vi "Periodic Tasks.vi"(8 "error in":errorcluster) -> ()   [LabVIEW 2015]
doc: "This VI runs in parallel to other tasks. It can contain as many user-defined periodic loops as you need. These can carry out PID or other sorts of timed response."
uses:
  Device Refnums.ctl
  Drive Base - Controlled Mode - TypeDef.ctl
  Drive Base Mode.ctl
  Shooter Control.ctl
  Arm Mode TypeDef.ctl
  <vilib>/Rock Robotics/WPI/Solenoid/WPI_SolenoidValue.ctl
  Projects/FRC Operator Interface Control Board/controlBoard_LabVIEW/LED_Output_TypeDef.ctl
  Projects/FRC Operator Interface Control Board/controlBoard_LabVIEW/PWM_Output_TypeDef.ctl
  <vilib>/Rock Robotics/WPI/CAN/TalonSRX/WPI_CANTalonSRX_APIControlMode.ctl
  <vilib>/Rock Robotics/WPI/Utilities/WPI_GetSetVariantRefNum.vi
  Global Variables.vi
  <vilib>/Rock Robotics/Network Tables/NT Write Number.vi
  <vilib>/Rock Robotics/Network Tables/NT Read Number.vi
  <vilib>/addons/control/pid/pid.llb/PID (DBL).vi
  <vilib>/Rock Robotics/Network Tables/NT Write Numeric Array.vi
  <vilib>/Rock Robotics/WPI/Solenoid/WPI_SolenoidSetEnum.vi
  <vilib>/Rock Robotics/Network Tables/NT Write String.vi
  <vilib>/Rock Robotics/Network Tables/NT Write Boolean.vi
  <vilib>/Rock Robotics/WPI/Ultrasonic/WPI_SonarMB1010DigitalRefNum Registry Get.vi
  <vilib>/Rock Robotics/WPI/Ultrasonic/WPI_SonarMB1010DigitalGetRange.vi
  ADIS16448-RoboRIO-Driver/trunk/LabVIEW/ADI MXP IMU/FRC ADI MXP IMU.lvlib
  <vilib>/addons/control/pid/NI_PID_pid.lvlib
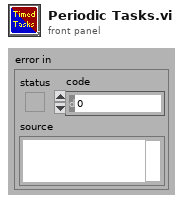
[diagram p1: front panel]
types:
  T1 = typedef "Device Refnums.ctl" = string
  T2 = typedef "Shooter Control.ctl" = cluster{"Fire":bool, "Open Claw":bool}
  T3 = typedef "Drive Base Mode.ctl" = enum16{"Disabled", "Controlled - Arcade", "Controlled - Tank", "Braked", "GRIP", "Encoder", "IMU", "Distance"}
  T4 = typedef "Drive Base - Controlled Mode - TypeDef.ctl" = cluster{"Drive Base Mode":T3, "Arcade":cluster{"y":dbl, "x":dbl}, "Tank":cluster{"Left":dbl, "Right":dbl}, "Target Encoder Value":cluster{"Left":dbl, "Right":dbl}, "Target IMU Angle":dbl, "Distance":dbl, "Target GRIP Area":dbl}
  T5 = typedef "WPI_EncoderDevRef.ctl" = cluster{"DevStatus":errorcluster, "EncoderIndex":T6, "CounterIndex":T7, "DistancePerCount":dbl, "Decoding Type":T8}
  T6 = typedef "FPGA_EncoderIdx.ctl" = enum8{"Enc 0", "Enc 1", "Enc 2", "Enc 3", "Enc 4", "Enc 5", "Enc 6", "Enc 7", "Invalid"}
  T7 = typedef "FPGA_CounterCtrSystemIndex.ctl" = enum8{"Ctr 0", "Ctr 1", "Ctr 2", "Ctr 3", "Ctr 4", "Ctr 5", "Ctr 6", "Ctr 7", "Invalid"}
  T8 = typedef "WPI_EncoderType.ctl" = enum16{"1x", "2x", "4x"}
  T9 = typedef "WPI_RobotDriveDevRef.ctl" = cluster{"DevStatus":errorcluster, "Motors[]":T10[], "Square Inputs":bool, "Max Output":dbl}
  T10 = typedef "WPI_MotorControlDeviceRef.ctl" = cluster{"DeviceStatus":errorcluster, "Type":T11, "PWM":cluster{"PWM Channel":T12, "DeadBand":T13}, "CAN":cluster{"Device Number":u8, "Control Mode":T14, "Semaphore":T15, "Max Vout":dbl, "TalonSRX Control Mode":T16}, "Invert":bool}
  T11 = typedef "WPI_MotorControlType.ctl" = enum16{"PWM", "CAN", "CANTalonSRX"}
  T12 = typedef "FPGA_DIOPWMChannel.ctl" = enum8{"PWM 0", "PWM 1", "PWM 2", "PWM 3", "PWM 4", "PWM 5", "PWM 6", "PWM 7", "PWM 8", "PWM 9", "PWM MXP 0", "PWM MXP 1", "PWM MXP 2", "PWM MXP 3", "PWM MXP 4", "PWM MXP 5", "PWM MXP 6", "PWM MXP 7", "PWM MXP 8", "PWM MXP 9", "Invalid"}
  T13 = typedef "WPI_PWMDeadband.ctl" = cluster{"Name":string, "maxPositivePwm":i32, "minPositivePwm":i32, "centerPwm":i32, "maxNegativePwm":i32, "minNegativePwm":i32, "angularRange":u16}
  T14 = typedef "WPI_CANJaguar_ControlMode.ctl" = enum8{"Percent VBus", "Current", "Speed", "Position", "Voltage"}
  T15 = typedef "Semaphore RefNum" = refnum<k1>
  T16 = typedef "WPI_CANTalonSRX_APIControlMode.ctl" = enum8{"Percent VBus", "Speed", "Position", "Slave", "Unchanged / Invalid", "Voltage Compensation", "Current", "Motion Profile"}
  T17 = typedef "WPI_SonarMB1010DigitalDeviceRef.ctl" = cluster{"CounterDevRef":T18, "Scaling factor (s/in)":dbl}
  T18 = typedef "WPI_CounterDevRef.ctl" = cluster{"DevStatus":errorcluster, "CntIndex":T7}
  T19 = typedef "FRC ADI MXP IMU.lvlib/WPI_AnalogDevicesIMUInterruptDevRef.ctl" = cluster{"SimpleGyroDevRef":T20, "InterruptRef":T22}
  T20 = typedef "FRC ADI MXP IMU.lvlib/WPI_AnalogDevicesIMUDevRef.ctl" = cluster{"DevStatus":errorcluster, "Handle":i32, "SPI Bus":T21, "Device Found":bool, "Sample Rate":dbl, "Device Ready":bool, "Yaw Axis":enum16{"X", "Y", "Z"}, "AHRS Algorithm":enum16{"Complementary", "Madgwick"}}
  T21 = typedef "spi_bus.ctl" = enum16{"SPI On-Board, CS0", "SPI On-Board, CS1", "SPI On-Board, CS2", "SPI On-Board, CS3", "SPI MXP", "Invalid"}
  T22 = typedef "WPI_InterruptRef.ctl" = cluster{"DevStatus":errorcluster, "InterruptIndex":T23}
  T23 = typedef "FPGA_InterruptIndex.ctl" = enum8{"0", "1", "2", "3", "4", "5", "6", "7", "Invalid"}
  T24 = typedef "WPI_AnalogChannelDevRef.ctl" = cluster{"DevStatus":errorcluster, "Analog Channel":T25}
  T25 = typedef "FPGA_AIChannel.ctl" = enum8{"AI 0", "AI 1", "AI 2", "AI 3", "AI MXP 0", "AI MXP 1", "AI MXP 2", "AI MXP 3", "Invalid"}
  T26 = typedef "Switch_Input_TypeDef.ctl" = cluster{"SW 0":bool, "SW 1":bool, "SW 2":bool, "SW 3":bool, "SW 4":bool, "SW 5":bool, "SW 6":bool, "SW 7":bool, "SW 8":bool, "SW 9":bool, "SW 10":bool, "SW 11":bool, "SW 12":bool, "SW 13":bool, "SW 14":bool, "SW 15":bool}
  T27 = typedef "GRIP Contours Report.ctl" = cluster{"area":dbl, "centerX":dbl, "centerY":dbl, "width":dbl, "height":dbl, "solidity":dbl}
  T28 = cluster{"proportional gain (Kc)":dbl, "integral time (Ti, min)":dbl, "derivative time (Td, min)":dbl}
  T29 = typedef "IMU AHRS TypeDef.ctl" = cluster{"Pitch":dbl, "Roll":dbl, "Yaw":dbl}
  T30 = typedef "WPI_SolenoidDevRef.ctl" = cluster{"DevStatus":errorcluster, "Pneumatics Control Module":u8, "Forward Solenoid Channel":T31, "Reverse Solenoid Channel":T31}
  T31 = typedef "WPI_SolenoidChannel.ctl" = enum8{"Solenoid 0", "Solenoid 1", "Solenoid 2", "Solenoid 3", "Solenoid 4", "Solenoid 5", "Solenoid 6", "Solenoid 7", "Invalid"}
  T32 = typedef "WPI_SolenoidValue.ctl" = enum16{"Off", "On", "Forward", "Reverse"}
  T33 = typedef "WPI_SwitchDevRef.ctl" = cluster{"DevStatus":errorcluster, "DIO Channel":T34, "CntIndex":T7, "Normally Closed":bool}
  T34 = typedef "FPGA_DIOChannel.ctl" = enum8{"DIO 0", "DIO 1", "DIO 2", "DIO 3", "DIO 4", "DIO 5", "DIO 6", "DIO 7", "DIO 8", "DIO 9", "DIO MXP 0", "DIO MXP 1", "DIO MXP 2", "DIO MXP 3", "DIO MXP 4", "DIO MXP 5", "DIO MXP 6", "DIO MXP 7", "DIO MXP 8", "DIO MXP 9", "DIO MXP 10", "DIO MXP 11", "DIO MXP 12", "DIO MXP 13", "DIO MXP 14", "DIO MXP 15", "Invalid"}
  T35 = typedef "Arm Mode TypeDef.ctl" = enum16{"Unknown", "Disabled", "Locked", "Shoot Batter", "Shoot Close", "Cross Defense", "Human Player Load", "Low Bar / Goal", "Manual"}
  T36 = typedef "Arm Notifier TypeDef.ctl" = cluster{"Arm Mode":T35, "Manual Arm Angle":dbl}
  T37 = typedef "PWM_Output_TypeDef.ctl" = cluster{"PWM 0":u8, "PWM 1":u8, "PWM 2":u8, "PWM 3":u8, "PWM 4":u8, "PWM 5":u8, "PWM 6":u8, "PWM 7":u8, "PWM 8":u8, "PWM 9":u8, "PWM 10":u8}
  T38 = typedef "LED_Output_TypeDef.ctl" = cluster{"LED 0":bool, "LED 1":bool, "LED 2":bool, "LED 3":bool, "LED 4":bool, "LED 5":bool, "LED 6":bool, "LED 7":bool, "LED 8":bool, "LED 9":bool, "LED 10":bool, "LED 11":bool, "LED 12":bool, "LED 13":bool, "LED 14":bool, "LED 15":bool}
  T39 = typedef "Arm Mode LEDs.ctl" = cluster{"Shoot Batter":bool, "Shoot Close":bool, "Shoot Far":bool, "Low Bar / Goal":bool, "Human Player Load":bool, "Manual":bool}
  T40 = typedef "Analog_Input_TypeDef.ctl" = cluster{"ANA 0":u8, "ANA 1":u8, "ANA 2":u8, "ANA 3":u8, "ANA 4":u8, "ANA 5":u8, "ANA 6":u8, "ANA 7":u8, "ANA 8":u8, "ANA 9":u8, "ANA 10":u8, "ANA 11":u8, "ANA 12":u8, "ANA 13":u8, "ANA 14":u8, "ANA 15":u8}
  T41 = typedef "Autonomous Mode.ctl" = enum16{"Off", "Cross Defense", "Shoot A/B", "Shoot C/D", "Shoot E"}
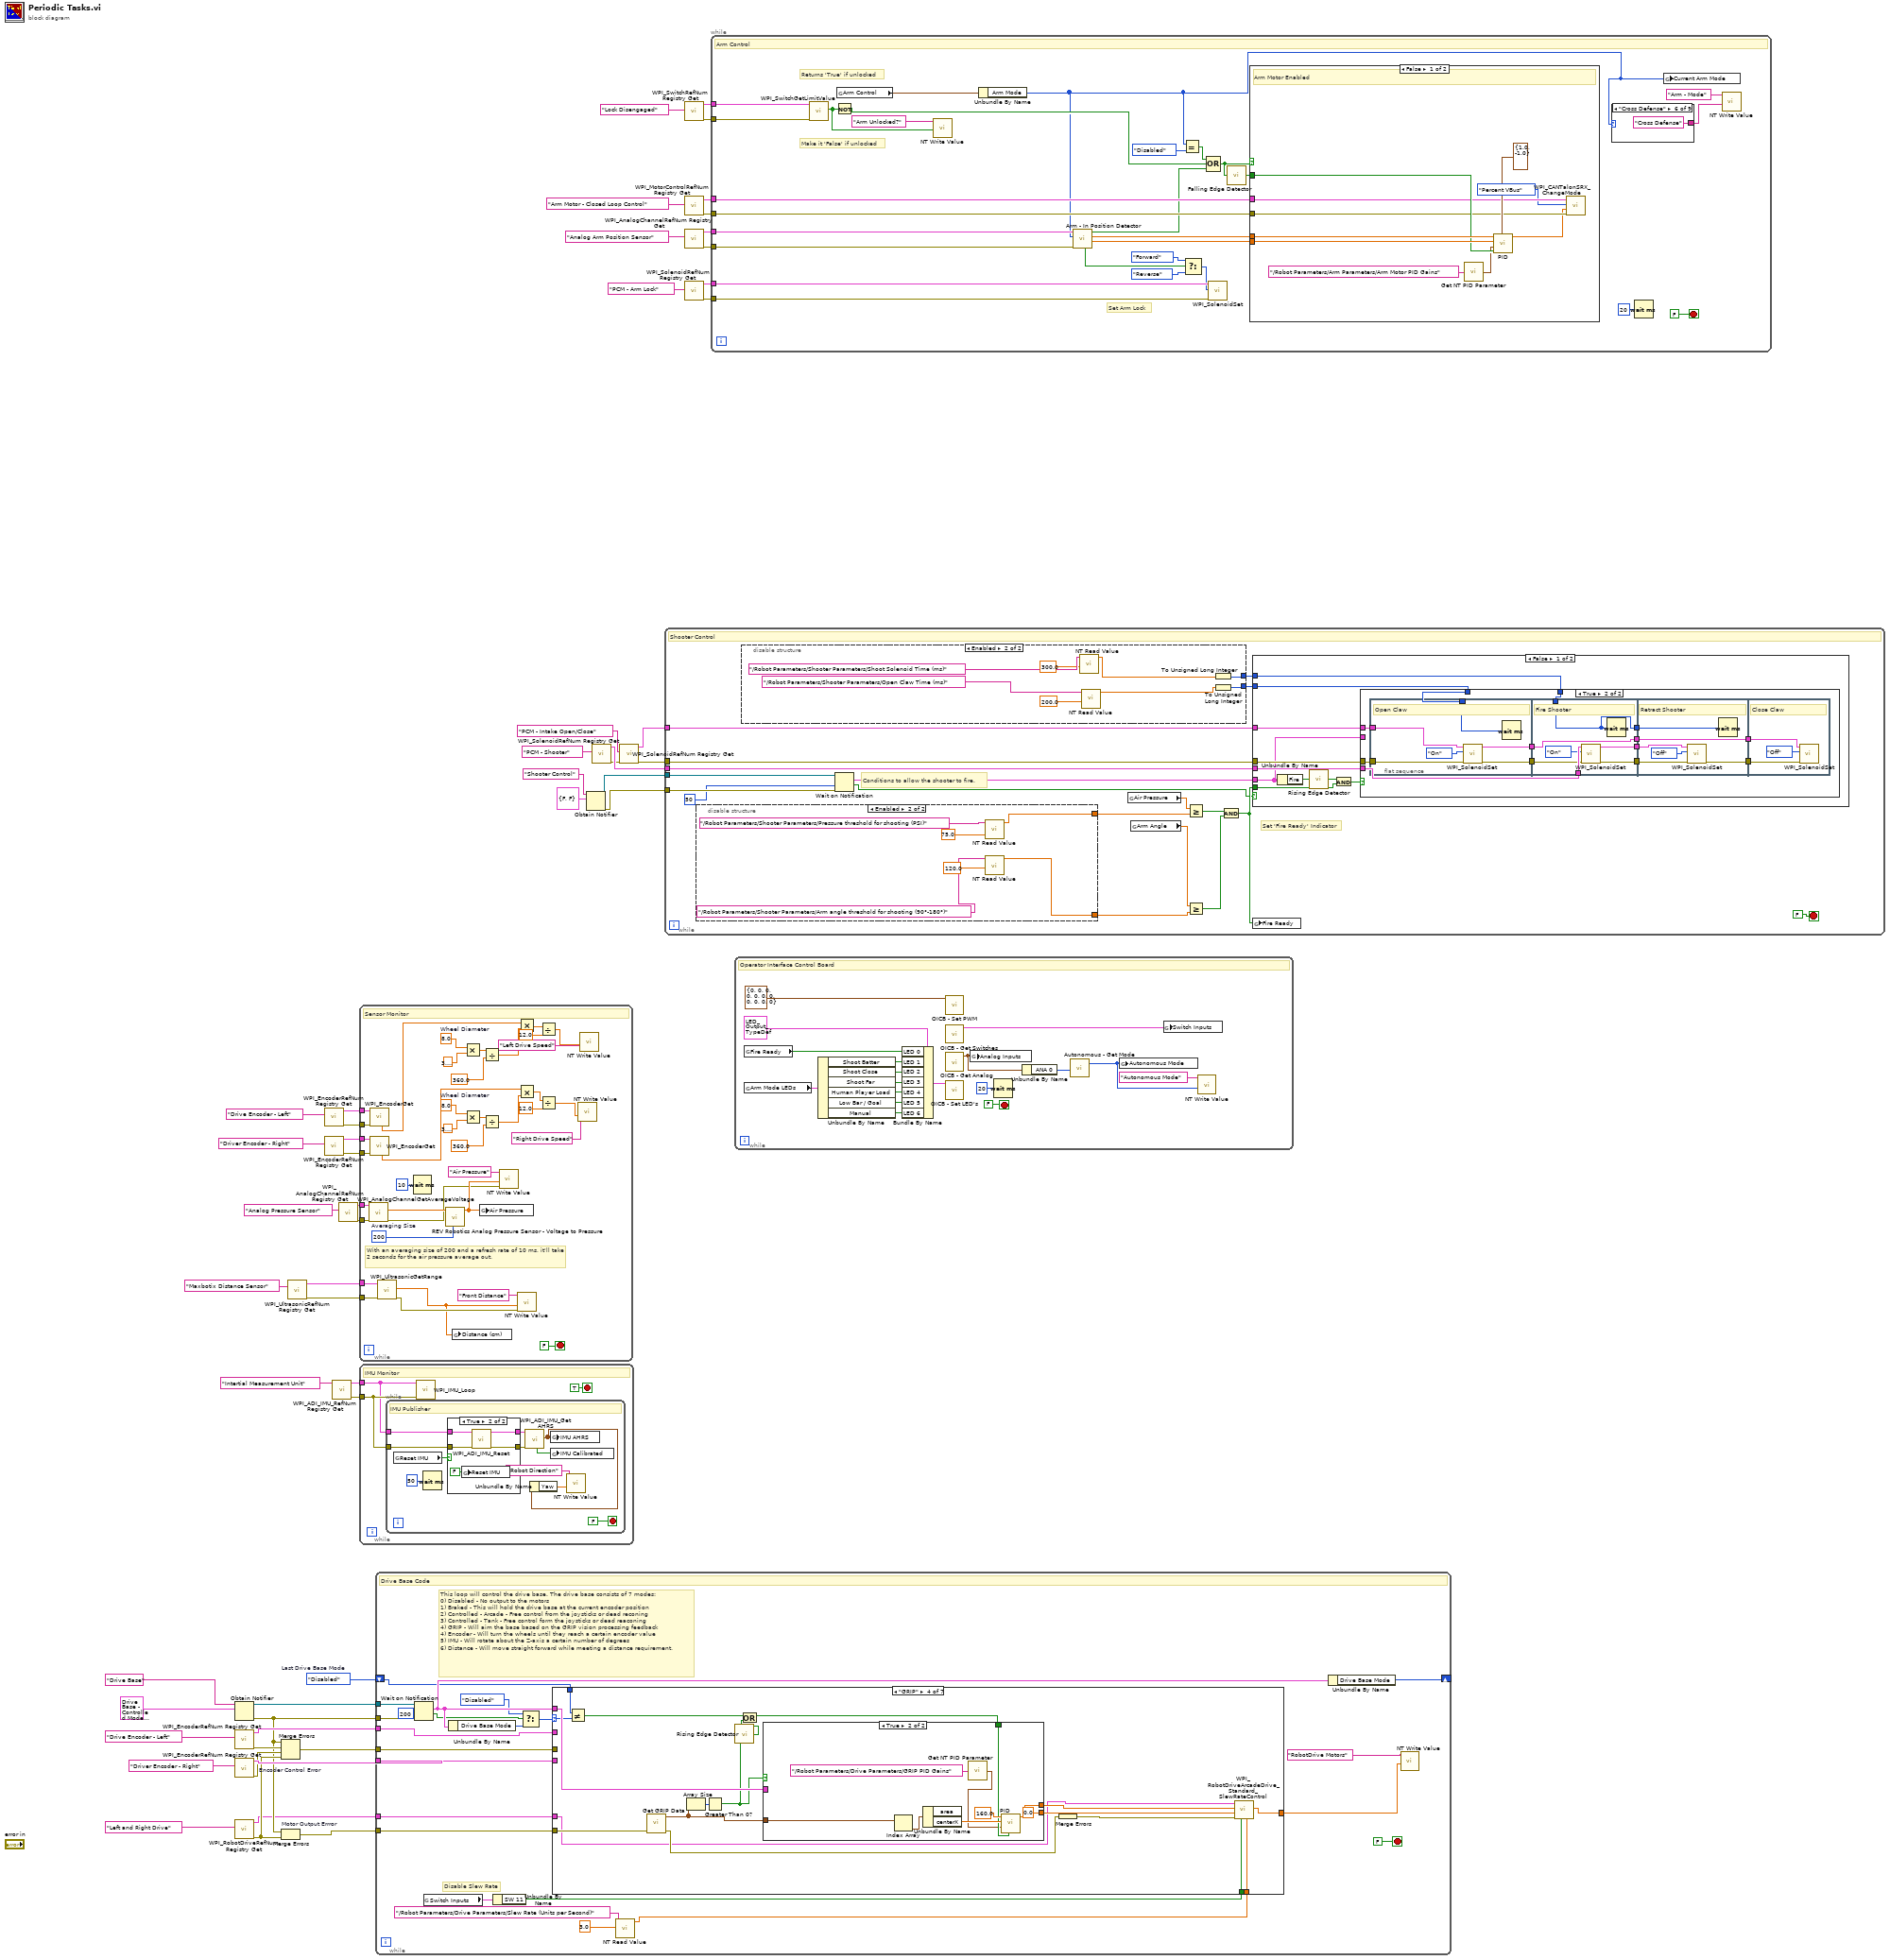
[diagram p0: block diagram]
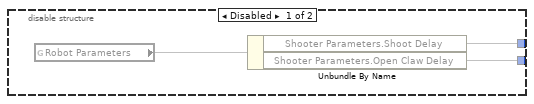
[diagram p3: hidden frame]
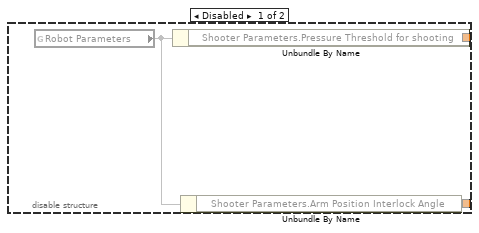
[diagram p4: hidden frame]
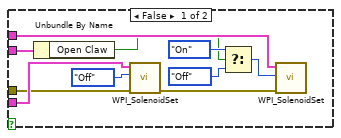
[diagram p5: hidden frame]
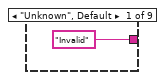
[diagram p7: hidden frame]
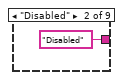
[diagram p8: hidden frame]
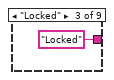
[diagram p9: hidden frame]
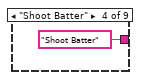
[diagram p10: hidden frame]
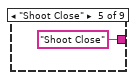
[diagram p11: hidden frame]
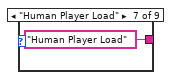
[diagram p12: hidden frame]
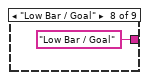
[diagram p13: hidden frame]
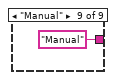
[diagram p14: hidden frame]
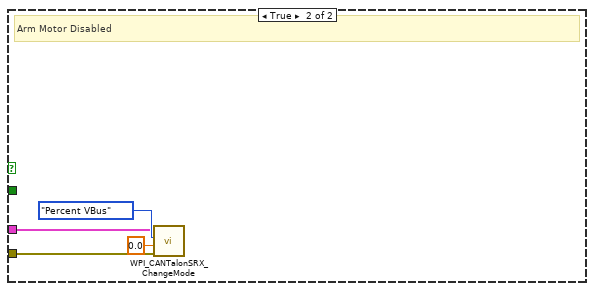
[diagram p15: hidden frame]
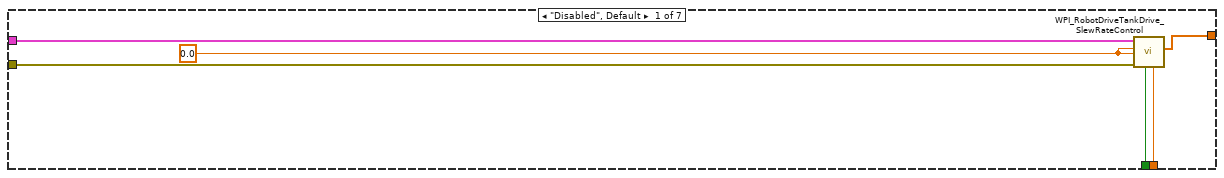
[diagram p16: hidden frame]
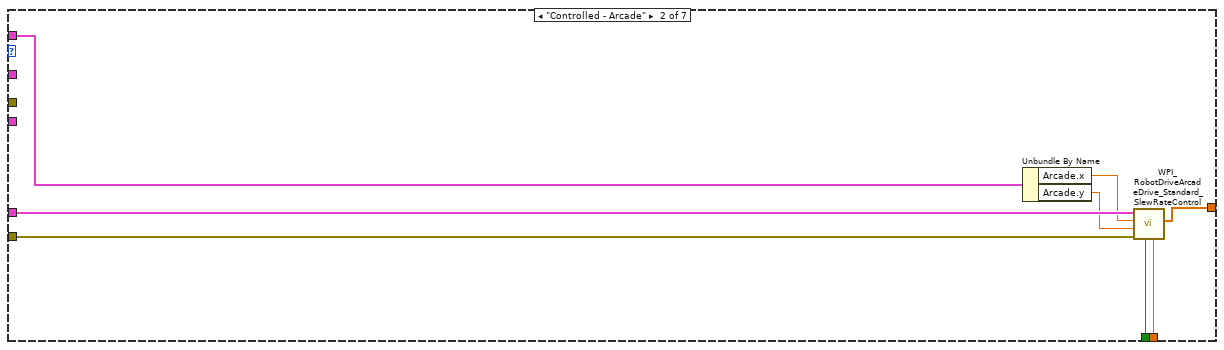
[diagram p17: hidden frame]
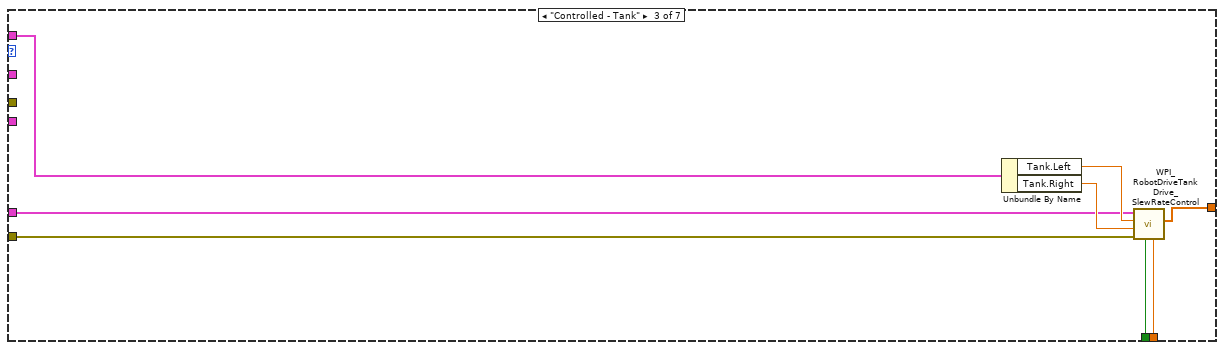
[diagram p18: hidden frame]
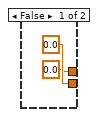
[diagram p19: hidden frame]
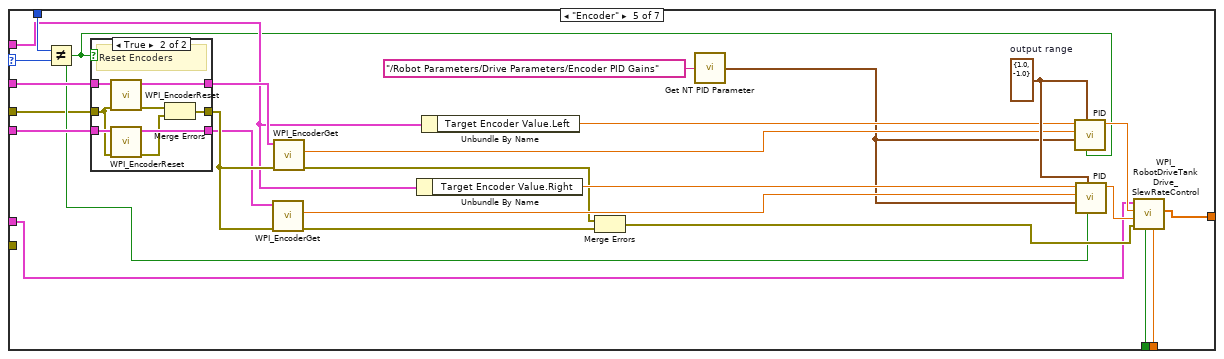
[diagram p20: hidden frame]
diagram:
  w37 = Drive_Base_Mode."Disabled"  # Last Drive Base Mode
  n1 = Obtain Notifier(name (unnamed)="Drive Base", notification data type=T4 {"Drive Base Mode"=enum."Disabled", "Arcade"={"y"=0.0, "x"=0.0}, "Tank"={"Left"=0.0, "Right"=0.0}, "Target Encoder Value"={"Left"=0.0, "Right"=0.0}, "Target IMU Angle"=0.0, "Distance"=0.0, "Target GRIP Area"=0.0}) -> (notifier out=w50:refnum<notifier>, error out=w40:errorcluster)  [unwired: 2 in, 1 out]
  n2 = call <vilib>:"WPI_EncoderRefNum Registry Get.vi"("refnum name"=T1 "Drive Encoder - Left" ("Device Name")) -> ("error out"=w44:errorcluster, "EncoderDevRef"=w47:T5)  [unwired: 9 in]
  n3 = call <vilib>:"WPI_EncoderRefNum Registry Get.vi"("refnum name"=T1 "Driver Encoder - Right" ("Device Name")) -> ("error out"=w43:errorcluster, "EncoderDevRef"=w46:T5)  [unwired: 9 in]
  n4 = call <vilib>:"WPI_RobotDriveRefNum Registry Get.vi"("refnum name"=T1 "Left and Right Drive" ("Device Name")) -> ("error out"=w41:errorcluster, "RobotDriveDevRef"=w39:T9)  [unwired: 1 in, 8 out]
  n5 = Merge Errors "Encoder Control Error"(w40, w44, w43, w41) -> (w42:errorcluster)
  n6 = Merge Errors "Motor Output Errror"(w40, w41) -> (w38:errorcluster)
  n7 = call-poly <vilib>:"WPI_UltrasonicRefNum Registry Get.vi"("refnum name"=T1 "Maxbotix Distance Sensor" ("Device Name")) -> ("error out"=w7:errorcluster, "SonarMB1010DigitalDevRef"=w8:T17)  [unwired: 9 in]
  n8 = call <vilib>:"WPI_EncoderRefNum Registry Get.vi"("refnum name"=T1 "Drive Encoder - Left" ("Device Name")) -> ("error out"=w3:errorcluster, "EncoderDevRef"=w4:T5)  [unwired: 9 in]
  n9 = call <vilib>:"WPI_EncoderRefNum Registry Get.vi"("refnum name"=T1 "Driver Encoder - Right" ("Device Name")) -> ("error out"=w1:errorcluster, "EncoderDevRef"=w2:T5)  [unwired: 9 in]
  n10 = call "WPI_ADI_IMU_RefNum Registry Get.vi"("refnum name"=T1 "Intertial Measurement Unit" ("Device Name")) -> ("error out"=w13:errorcluster, "ADI IMU Interrupt DevRef"=w12:T19)  [unwired: 9 in]
  n11 = call <vilib>:"WPI_AnalogChannelRefNum Registry Get.vi"("refnum name"=T1 "Analog Pressure Sensor" ("Device Name")) -> ("error out"=w18:errorcluster, "AIDeviceRef"=w19:T24)  [unwired: 9 in]
  n12 = while {
    tunnel: w19 -> [w87]
    tunnel: w18 -> [w86]
    tunnel: w8 -> [w82]
    tunnel: w7 -> [w83]
    tunnel: w4 -> [w77]
    tunnel: w3 -> [w76]
    tunnel: w2 -> [w75]
    tunnel: w1 -> [w74]
    stop <- FALSE stop-if-true
    w67 = 8.0  # Wheel Diameter
    w70 = 8.0  # Wheel Diameter
    w85 = 200  # Averaging Size
    # "With an averaging size of 200 and a refresh rate of 10 ms, it'll take 2 seconds for the air pressure average out."
    # "Sensor Monitor"
    n13 = call <vilib>:"WPI_AnalogChannelGetAverageVoltage.vi"("error in (no error)"=w86, "AIDeviceRef"=w87) -> ("error out"=w79:errorcluster, "Voltage"=w89:dbl)  [unwired: 7 in, 1 out]
    n14 = call <vilib>:"WPI_EncoderGet.vi"("error in (no error)"=w76, "EncoderDevRef"=w77) -> ("Rate"=w63:dbl)  [unwired: 4 in, 5 out]
    n15 = call <vilib>:"WPI_EncoderGet.vi"("error in (no error)"=w74, "EncoderDevRef"=w75) -> ("Rate"=w62:dbl)  [unwired: 4 in, 5 out]
    n16 = call-poly <vilib>:"WPI_UltrasonicGetRange.vi"("error in"=w83, "SonarMB1010DigitalDevRef"=w82) -> ("error out"=w80:errorcluster, "Distance"=w78:dbl)  [unwired: 7 in, 1 out]
    n17 = Wait (ms)(milliseconds to wait=u32 10) -> ()  [unwired: 1 out]
    n18 = call "REV Robotics Analog Pressure Sensor - Voltage to Pressure.vi"("Averaging Size"=w85, "Voltage (V)"=w89) -> ("Pressure (PSI)"=w84:dbl)  [unwired: 7 in]
    n19 = global write "Global Variables.vi" "Distance (cm)"(w78) -> ()
    n20 = Multiply(x=w67, y=3.141592653589793) -> (x*y=w66:dbl)
    n21 = Multiply(x=w70, y=3.141592653589793) -> (x*y=w71:dbl)
    n22 = global write "Global Variables.vi" "Air Pressure"(w84) -> ()
    n23 = Divide(x=w66, y=360.0) -> (x/y=w64:dbl)
    n24 = Divide(x=w71, y=360.0) -> (x/y=w73:dbl)
    n25 = call-poly <vilib>:"NT Write Value.vi"("error in"=w79, "Numeric"=w84, "Name"="Air Pressure") -> ()  [unwired: 8 in, 1 out]
    n26 = call-poly <vilib>:"NT Write Value.vi"("error in"=w80, "Numeric"=w78, "Name"="Front Distance") -> ()  [unwired: 8 in, 1 out]
    n27 = Multiply(x=w63, y=w64) -> (x*y=w61:dbl)
    n28 = Multiply(x=w62, y=w73) -> (x*y=w58:dbl)
    n29 = Divide(x=w61, y=12.0) -> (x/y=w54:dbl)
    n30 = Divide(x=w58, y=12.0) -> (x/y=w55:dbl)
    n31 = call-poly <vilib>:"NT Write Value.vi"("Numeric"=w55, "Name"="Right Drive Speed") -> ()  [unwired: 9 in, 1 out]
    n32 = call-poly <vilib>:"NT Write Value.vi"("Numeric"=w54, "Name"="Left Drive Speed") -> ()  [unwired: 9 in, 1 out]
  }
  n33 = while {
    tunnel: w13 -> [w94]
    tunnel: w12 -> [w93]
    stop <- TRUE stop-if-true
    # "IMU Monitor"
    n34 = while {
      tunnel: w94 -> [w101]
      tunnel: w93 -> [w102]
      stop <- FALSE stop-if-true
      # "IMU Publisher"
      n35 = global read "Global Variables.vi" "Reset IMU"() -> (w103:bool)
      n36 = Wait (ms)(milliseconds to wait=u32 50) -> ()  [unwired: 1 out]
      n37 = case shown="True" w103 {
        tunnel: w102 -> [w107 w111]
        tunnel: w101 -> [w106 w110]
        tunnel: [w107 w109] -> w99
        tunnel: [w106 w108] -> w98
        frame False {
        }
        frame True {
          n38 = global write "Global Variables.vi" "Reset IMU"(FALSE ("Reset IMU")) -> ()
          n39 = call "WPI_ADI_IMU_Reset.vi"("error in"=w110, "ADI IMU Interrupt DevRef"=w111) -> ("error out"=w108:errorcluster, "ADI IMU Interrupt DevRef Out"=w109:T19)  [unwired: 8 in]
        }
      }
      n40 = call "WPI_ADI_IMU_Get AHRS.vi"("error in"=w98, "ADI IMU Interrupt DevRef"=w99) -> ("IMU AHRS"=w96:cluster{"Pitch":dbl, "Roll":dbl, "Yaw":dbl}, "Sensor Ready Out"=w100:bool)  [unwired: 5 in, 3 out]
      n41 = Unbundle By Name(w96) -> ("Yaw"=w95:dbl)
      n42 = global write "Global Variables.vi" "IMU AHRS"(w96) -> ()
      n43 = global write "Global Variables.vi" "IMU Calibrated"(w100) -> ()
      n44 = call-poly <vilib>:"NT Write Value.vi"("Numeric"=w95, "Name"="Robot Direction") -> ()  [unwired: 9 in, 1 out]
    }
    n45 = call "WPI_IMU_Loop.vi"("error in"=w94, "ADI IMU Interrupt DevRef"=w93) -> ()  [unwired: 8 in, 2 out]
  }
  n46 = while {
    tunnel: w39 -> [w134]
    tunnel: w50 -> [w133]
    tunnel: w40 -> [w132]
    tunnel: w47 -> [w131]
    tunnel: w46 -> [w130]
    tunnel: w42 -> [w128]
    tunnel: w38 -> [w129]
    shift-right: [w127] -> _
    shift-left: w37 -> [w125]
    stop <- FALSE stop-if-true
    # "Disable Slew Rate"
    # "This loop will control the drive base. The drive base consists of 7 modes:\n0) Disabled - No output to the motors\n1) Braked - This will hold the drive base at the current encoder position\n2) Controlled - Arcade - Free control from the joysticks or dead reconing\n3) Controlled - Tank - Free control form the joysticks or dead reaconing\n4) GRIP - Will aim the base based on the GRIP vision processing feedback\n4) Encoder - Will turn the wheels until they reach a certain encoder value\n5) IMU - Will rotate about the Z-axis a certain number of degrees\n6) Distance - Will move straight forward while meeting a distance requirement."
    # "Drive Base Code"
    n47 = Wait on Notification(notifier=w133, timeout in ms (-1)=200, error in (no error)=w132) -> (notification=w126:T4, timed out?=w123:bool)  [unwired: 1 in, 2 out]
    n48 = global read "Global Variables.vi" "Switch Inputs"() -> (w117:T26)
    n49 = Unbundle By Name(w126) -> ("Drive Base Mode"=w122:T3)
    n50 = Unbundle By Name(w117) -> ("SW 11"=w116:bool)
    n51 = Select(t=Drive_Base_Mode."Disabled", s=w123, f=w122) -> (s? t:f=w120:T3)
    n52 = call-poly <vilib>:"NT Read Value.vi"("Default Value"=3.0, "Name"="/Robot Parameters/Drive Parameters/Slew Rate (Units per Second)") -> ("Numeric"=w115:dbl)  [unwired: 8 in, 1 out]
    n53 = case shown="\"GRIP\"" w120 {
      selector: w120 -> [_ _ _ w172 w211 w241 w260]
      tunnel: w134 -> [w141 w149 w154 w160 w194 w238 w259]
      tunnel: w126 -> [_ w147 w153 w175 w198 w237 _]
      tunnel: w131 -> [_ _ _ _ w210 _ w265]
      tunnel: w130 -> [_ _ _ _ w209 _ w264]
      tunnel: w129 -> [w139 w148 w155 w174 _ w236 _]
      tunnel: w128 -> [_ _ _ _ w191 _ w257]
      tunnel: w125 -> [_ _ _ w171 w212 w240 w261]
      tunnel: [w138 w144 w152 w164 w193 w231 w258] -> w118
      tunnel: w116 -> [w137 w143 w151 w159 w190 w227 w256]
      tunnel: w115 -> [w136 w142 w150 w158 w189 w226 w255]
      frame "Disabled", Default {
        w140 = 0.0
        n54 = call "WPI_RobotDriveTankDrive_SlewRateControl.vi"("Slew Rate (Unit/Sec)"=w136, "Disable Slew"=w137, "error in (no error)"=w139, "Right axis value"=w140, "Left axis value"=w140, "RobotDriveDevRef"=w141) -> ("Motor Values"=w138:dbl[])  [unwired: 3 in, 2 out]
      }
      frame "Controlled - Arcade" {
        n55 = Unbundle By Name(w147) -> ("Arcade.x"=w145:dbl, "Arcade.y"=w146:dbl)
        n56 = call "WPI_RobotDriveArcadeDrive_Standard_SlewRateControl.vi"("Slew Rate (Unit/Sec)"=w142, "Disable Slew"=w143, "error in (no error)"=w148, "Y axis value"=w146, "X axis value"=w145, "RobotDriveDevRef"=w149) -> ("Motor Values"=w144:dbl[])  [unwired: 3 in, 2 out]
      }
      frame "Controlled - Tank" {
        n57 = Unbundle By Name(w153) -> ("Tank.Left"=w157:dbl, "Tank.Right"=w156:dbl)
        n58 = call "WPI_RobotDriveTankDrive_SlewRateControl.vi"("Slew Rate (Unit/Sec)"=w150, "Disable Slew"=w151, "error in (no error)"=w155, "Right axis value"=w156, "Left axis value"=w157, "RobotDriveDevRef"=w154) -> ("Motor Values"=w152:dbl[])  [unwired: 3 in, 2 out]
      }
      frame "GRIP" {
        n59 = Not Equal?(x=w171, y=w172) -> (x != y?=w170:bool)
        n60 = call "Get GRIP Data.vi"("error in (no error)"=w174) -> ("error out"=w173:errorcluster, "ContoursReport"=w169:T27[])  [unwired: 8 in, 1 out]
        n61 = Array Size(array=w169) -> (size(s)=w168:i32)
        n62 = Greater Than 0?(x=w168) -> (x > 0?=w167:bool)
        n63 = call "Rising Edge Detector.vi"("Input"=w167) -> ("Rising Edge Detected"=w165:bool)
        n64 = Or(x=w170, y=w165) -> (x .or. y?=w166:bool)
        n65 = case shown="True" w167 {
          tunnel: w175 -> [_ _]
          tunnel: w166 -> [_ w183]
          tunnel: [0.0 ("output") 0.0 ("output")] -> w162
          tunnel: [0.0 ("output") w182] -> w163
          tunnel: w169 -> [_ w181]
          frame False {
          }
          frame True {
            n66 = Index Array(array=w181) -> (element=w186:T27)  [unwired: 1 in]
            n67 = Unbundle By Name(w186) -> ("centerX"=w185:dbl)  [unwired: 1 out]
            n68 = call "Get NT PID Parameter.vi"("NT Path"="/Robot Parameters/Drive Parameters/GRIP PID Gains") -> ("PID Gains"=w178:T28)
            n69 = call-poly <vilib>:"PID.vi"("reinitialize? (F)"=w183, "PID gains"=w178, "process variable"=w185, "setpoint"=160.0) -> ("output"=w182:dbl)  [unwired: 6 in, 1 out]
          }
        }
        n70 = Merge Errors(w173) -> (w161:errorcluster)
        n71 = call "WPI_RobotDriveArcadeDrive_Standard_SlewRateControl.vi"("Slew Rate (Unit/Sec)"=w158, "Disable Slew"=w159, "error in (no error)"=w161, "Y axis value"=w162, "X axis value"=w163, "RobotDriveDevRef"=w160) -> ("Motor Values"=w164:dbl[])  [unwired: 3 in, 2 out]
      }
      frame "Encoder" {
        w208 = cluster{"output high":dbl, "output low":dbl} {"output high"=1.0, "output low"=-1.0}  # output range
        n72 = Not Equal?(x=w212, y=w211) -> (x != y?=w192:bool)
        n73 = case shown="True" w192 {
          tunnel: w210 -> [w215 w223]
          tunnel: w209 -> [w214 w222]
          tunnel: [w215 w221] -> w206
          tunnel: [w214 w220] -> w205
          tunnel: [w213 w219] -> w207
          tunnel: w191 -> [w213 w216]
          frame False {
          }
          frame True {
            # "Reset Encoders"
            n74 = call <vilib>:"WPI_EncoderReset.vi"("error in (no error)"=w216, "EncoderDevRef"=w223) -> ("error out"=w218:errorcluster, "EncoderDevRef"=w221:T5)  [unwired: 8 in]
            n75 = call <vilib>:"WPI_EncoderReset.vi"("error in (no error)"=w216, "EncoderDevRef"=w222) -> ("error out"=w217:errorcluster, "EncoderDevRef"=w220:T5)  [unwired: 8 in]
            n76 = Merge Errors(w218, w217) -> (w219:errorcluster)
          }
        }
        n77 = call <vilib>:"WPI_EncoderGet.vi"("error in (no error)"=w207, "EncoderDevRef"=w205) -> ("error out"=w196:errorcluster, "Distance"=w203:dbl)  [unwired: 4 in, 4 out]
        n78 = call <vilib>:"WPI_EncoderGet.vi"("error in (no error)"=w207, "EncoderDevRef"=w206) -> ("error out"=w197:errorcluster, "Distance"=w204:dbl)  [unwired: 4 in, 4 out]
        n79 = Unbundle By Name(w198) -> ("Target Encoder Value.Right"=w199:dbl)
        n80 = Unbundle By Name(w198) -> ("Target Encoder Value.Left"=w200:dbl)
        n81 = Merge Errors(w197, w196) -> (w195:errorcluster)
        n82 = call "Get NT PID Parameter.vi"("NT Path"="/Robot Parameters/Drive Parameters/Encoder PID Gains") -> ("PID Gains"=w187:T28)
        n83 = call-poly <vilib>:"PID.vi"("reinitialize? (F)"=w192, "output range"=w208, "PID gains"=w187, "process variable"=w204, "setpoint"=w200) -> ("output"=w202:dbl)  [unwired: 5 in, 1 out]
        n84 = call-poly <vilib>:"PID.vi"("reinitialize? (F)"=w192, "output range"=w208, "PID gains"=w187, "process variable"=w203, "setpoint"=w199) -> ("output"=w201:dbl)  [unwired: 5 in, 1 out]
        n85 = call "WPI_RobotDriveTankDrive_SlewRateControl.vi"("Slew Rate (Unit/Sec)"=w189, "Disable Slew"=w190, "error in (no error)"=w195, "Right axis value"=w201, "Left axis value"=w202, "RobotDriveDevRef"=w194) -> ("Motor Values"=w193:dbl[])  [unwired: 3 in, 2 out]
      }
      frame "IMU" {
        n86 = Not Equal?(x=w240, y=w241) -> (x != y?=w230:bool)
        n87 = global read "Global Variables.vi" "IMU AHRS"() -> (w229:T29)
        n88 = global read "Global Variables.vi" "IMU Calibrated"() -> (w228:bool)
        n89 = global write "Global Variables.vi" "Reset IMU"(w230) -> ()
        n90 = call "Get NT PID Parameter.vi"("NT Path"="/Robot Parameters/Drive Parameters/IMU PID Gains") -> ("PID Gains"=w224:T28)
        n91 = Not(x=w230) -> (.not. x?=w234:bool)
        n92 = And(x=w228, y=w234) -> (x .and. y?=w233:bool)
        n93 = feedback-in #1(w233) -> ()
        n94 = feedback #1() -> (w232:bool)  [unwired: 1 in]
        n95 = case shown="True" w233 {
          selector: w233 -> [_ w247]
          tunnel: w229 -> [_ w252]
          tunnel: w237 -> [_ w250]
          tunnel: [0.0 ("Y axis value") w244] -> w235
          tunnel: w232 -> [_ w248]
          tunnel: w224 -> [_ w243]
          frame False {
          }
          frame True {
            w245 = cluster{"output high":dbl, "output low":dbl} {"output high"=1.0, "output low"=-1.0}  # output range
            n96 = Unbundle By Name(w250) -> ("Target IMU Angle"=w249:dbl)
            n97 = Unbundle By Name(w252) -> ("Yaw"=w251:dbl)
            n98 = Greater?(x=w247, y=w248) -> (0:w246:bool)
            n99 = call-poly <vilib>:"PID.vi"("reinitialize? (F)"=w246, "output range"=w245, "PID gains"=w243, "process variable"=w251, "setpoint"=w249) -> ("output"=w244:dbl)  [unwired: 5 in, 1 out]
          }
        }
        n100 = call "WPI_RobotDriveArcadeDrive_Standard_SlewRateControl.vi"("Slew Rate (Unit/Sec)"=w226, "Disable Slew"=w227, "error in (no error)"=w236, "Y axis value"=0.0, "X axis value"=w235, "RobotDriveDevRef"=w238) -> ("Motor Values"=w231:dbl[])  [unwired: 3 in, 2 out]
      }
      frame "Braked" {
        w277 = cluster{"output high":dbl, "output low":dbl} {"output high"=1.0, "output low"=-1.0}  # output range
        n101 = Not Equal?(x=w261, y=w260) -> (x != y?=w275:bool)
        n102 = case shown="True" w275 {
          tunnel: [w280 w288] -> w274
          tunnel: [w279 w287] -> w273
          tunnel: [w278 w286] -> w276
          tunnel: w265 -> [w280 w283]
          tunnel: w264 -> [w279 w282]
          tunnel: w257 -> [w278 w281]
          frame False {
          }
          frame True {
            # "Reset Encoders"
            n103 = call <vilib>:"WPI_EncoderReset.vi"("error in (no error)"=w281, "EncoderDevRef"=w283) -> ("error out"=w285:errorcluster, "EncoderDevRef"=w288:T5)  [unwired: 8 in]
            n104 = call <vilib>:"WPI_EncoderReset.vi"("error in (no error)"=w281, "EncoderDevRef"=w282) -> ("error out"=w284:errorcluster, "EncoderDevRef"=w287:T5)  [unwired: 8 in]
            n105 = Merge Errors(w285, w284) -> (w286:errorcluster)
          }
        }
        n106 = call "Get NT PID Parameter.vi"("NT Path"="/Robot Parameters/Drive Parameters/Encoder PID Gains") -> ("PID Gains"=w254:T28)
        n107 = call <vilib>:"WPI_EncoderGet.vi"("error in (no error)"=w276, "EncoderDevRef"=w273) -> ("error out"=w267:errorcluster, "Distance"=w271:dbl)  [unwired: 4 in, 4 out]
        n108 = call <vilib>:"WPI_EncoderGet.vi"("error in (no error)"=w276, "EncoderDevRef"=w274) -> ("error out"=w268:errorcluster, "Distance"=w272:dbl)  [unwired: 4 in, 4 out]
        n109 = Merge Errors(w268, w267) -> (w266:errorcluster)
        n110 = call-poly <vilib>:"PID.vi"("reinitialize? (F)"=w275, "output range"=w277, "PID gains"=w254, "process variable"=w272, "setpoint"=0.0) -> ("output"=w270:dbl)  [unwired: 5 in, 1 out]
        n111 = call-poly <vilib>:"PID.vi"("reinitialize? (F)"=w275, "output range"=w277, "PID gains"=w254, "process variable"=w271, "setpoint"=0.0) -> ("output"=w269:dbl)  [unwired: 5 in, 1 out]
        n112 = call "WPI_RobotDriveTankDrive_SlewRateControl.vi"("Slew Rate (Unit/Sec)"=w255, "Disable Slew"=w256, "error in (no error)"=w266, "Right axis value"=w269, "Left axis value"=w270, "RobotDriveDevRef"=w259) -> ("Motor Values"=w258:dbl[])  [unwired: 3 in, 2 out]
      }
    }
    n113 = Unbundle By Name(w126) -> ("Drive Base Mode"=w127:T3)
    n114 = call-poly <vilib>:"NT Write Value.vi"("Numeric Array"=w118, "Name"="RobotDrive Motors") -> ()  [unwired: 9 in, 1 out]
  }
  n115 = Obtain Notifier(name (unnamed)="Shooter Control", notification data type=T2 {"Fire"=FALSE, "Open Claw"=FALSE}) -> (notifier out=w17:refnum<notifier>, error out=w16:errorcluster)  [unwired: 2 in, 1 out]
  n116 = call <vilib>:"WPI_SolenoidRefNum Registry Get.vi"("refnum name"=T1 "PCM - Shooter" ("Device Name")) -> ("error out"=w20:errorcluster, "SolenoidDevRef"=w21:T30)  [unwired: 9 in]
  n117 = call <vilib>:"WPI_SolenoidRefNum Registry Get.vi"("error in (no error)"=w20, "refnum name"=T1 "PCM - Intake Open/Close" ("Device Name")) -> ("error out"=w23:errorcluster, "SolenoidDevRef"=w24:T30)  [unwired: 8 in]
  n118 = while {
    tunnel: w24 -> [w305]
    tunnel: w23 -> [w304]
    tunnel: w21 -> [w303]
    tunnel: w17 -> [w301]
    tunnel: w16 -> [w300]
    stop <- FALSE ("stop") stop-if-true
    # "Set 'Fire Ready' Indicator"
    # "Conditions to allow the shooter to fire."
    # "Shooter Control"
    n119 = disable-structure shown="Enabled" {
      disable-tunnel: [w320 w325] -> w295
      disable-tunnel: [w318 w321] -> w290
      frame Disabled {
        n120 = global read "Global Variables.vi" "Robot Parameters"() -> (w319)
        n121 = Unbundle By Name(w319) -> ("Shooter Parameters.Pressure Threshold for shooting"=w320)
        n122 = Unbundle By Name(w319) -> ("Shooter Parameters.Arm Position Interlock Angle"=w318)
      }
      frame Enabled {
        n123 = call-poly <vilib>:"NT Read Value.vi"("Default Value"=75.0, "Name"="/Robot Parameters/Shooter Parameters/Pressure threshold for shooting (PSI)") -> ("Numeric"=w325:dbl)  [unwired: 8 in, 1 out]
        n124 = call-poly <vilib>:"NT Read Value.vi"("Default Value"=120.0, "Name"="/Robot Parameters/Shooter Parameters/Arm angle threshold for shooting (90°-180°)") -> ("Numeric"=w321:dbl)  [unwired: 8 in, 1 out]
      }
    }
    n125 = disable-structure shown="Enabled" {
      disable-tunnel: [w308 w312] -> w294
      disable-tunnel: [w307 w311] -> w293
      frame Disabled {
        n126 = global read "Global Variables.vi" "Robot Parameters"() -> (w309)
        n127 = Unbundle By Name(w309) -> ("Shooter Parameters.Shoot Delay"=w307, "Shooter Parameters.Open Claw Delay"=w308)
      }
      frame Enabled {
        n128 = call-poly <vilib>:"NT Read Value.vi"("Default Value"=300.0, "Name"="/Robot Parameters/Shooter Parameters/Shoot Solenoid Time (ms)") -> ("Numeric"=w313:dbl)  [unwired: 8 in, 1 out]
        n129 = call-poly <vilib>:"NT Read Value.vi"("Default Value"=200.0, "Name"="/Robot Parameters/Shooter Parameters/Open Claw Time (ms)") -> ("Numeric"=w310:dbl)  [unwired: 8 in, 1 out]
        n130 = To Unsigned Long Integer(number=w313) -> (unsigned 32bit integer=w311:u32)
        n131 = To Unsigned Long Integer(number=w310) -> (unsigned 32bit integer=w312:u32)
      }
    }
    n132 = Wait on Notification(notifier=w301, timeout in ms (-1)=50, error in (no error)=w300) -> (notification=w297:T2, timed out?=w296:bool)  [unwired: 1 in, 2 out]
    n133 = global read "Global Variables.vi" "Air Pressure"() -> (w302:dbl)
    n134 = global read "Global Variables.vi" "Arm Angle"() -> (w291:dbl)
    n135 = Greater Or Equal?(x=w302, y=w295) -> (x >= y?=w292:bool)
    n136 = Greater Or Equal?(x=w291, y=w290) -> (x >= y?=w289:bool)
    n137 = Compound Arithmetic op=AND(w292, w289) -> (w299:bool)
    n138 = case shown="False" w296 {
      tunnel: w305 -> [w335 _]
      tunnel: w304 -> [w334 _]
      tunnel: w303 -> [w333 _]
      tunnel: w299 -> [w331 _]
      tunnel: w297 -> [w329 _]
      tunnel: w294 -> [w328 _]
      tunnel: w293 -> [w327 _]
      frame False {
        n139 = Unbundle By Name(w329) -> ("Fire"=w330:bool)
        n140 = call "Rising Edge Detector.vi"("Input"=w330) -> ("Rising Edge Detected"=w332:bool)
        n141 = And(x=w332, y=w331) -> (x .and. y?=w336:bool)
        n142 = case shown="True" w336 {
          tunnel: w335 -> [w346 w359]
          tunnel: w334 -> [w343 w358]
          tunnel: w333 -> [w344 w357]
          tunnel: w329 -> [w341 _]
          tunnel: w328 -> [_ w349]
          tunnel: w327 -> [_ w348]
          frame False {
            n143 = Unbundle By Name(w341) -> ("Open Claw"=w337:bool)
            n144 = call-poly <vilib>:"WPI_SolenoidSet.vi"("error in (no error)"=w343, "Value"=WPI_SolenoidValue."Off", "SolenoidDevRef"=w344) -> ("error out"=w342:errorcluster)  [unwired: 7 in, 1 out]
            n145 = Select(t=WPI_SolenoidValue."On" ("Value"), s=w337, f=WPI_SolenoidValue."Off" ("Value")) -> (s? t:f=w340:T32)
            n146 = call-poly <vilib>:"WPI_SolenoidSet.vi"("error in (no error)"=w342, "Value"=w340, "SolenoidDevRef"=w346) -> ()  [unwired: 7 in, 2 out]
          }
          frame True {
            n147 = flat-sequence {
              tunnel: w359 -> [w365]
              tunnel: w358 -> [w364]
              tunnel: [w363] -> w355
              tunnel: [w362] -> w353
              tunnel: w349 -> [w360]
              tunnel: w357 -> [w372]
              tunnel: [w371] -> w356
              tunnel: w355 -> [w370]
              tunnel: [w370] -> w354
              tunnel: w353 -> [w369]
              tunnel: [w368] -> w352
              tunnel: w348 -> [w366]
              tunnel: [w366] -> w347
              tunnel: w356 -> [w378]
              tunnel: w354 -> [w374]
              tunnel: w352 -> [w377]
              tunnel: [w376] -> w351
              tunnel: [w374] -> w350
              tunnel: w347 -> [w373]
              tunnel: w351 -> [w381]
              tunnel: w350 -> [w379]
              frame #0 {
                # "Open Claw"
                n148 = call-poly <vilib>:"WPI_SolenoidSet.vi"("error in (no error)"=w364, "Value"=WPI_SolenoidValue."On", "SolenoidDevRef"=w365) -> ("error out"=w362:errorcluster, "SolenoidDevRef"=w363:T30)  [unwired: 7 in]
                n149 = Wait (ms)(milliseconds to wait=w360) -> ()  [unwired: 1 out]
              }
              frame #1 {
                # "Fire Shooter"
                n150 = call-poly <vilib>:"WPI_SolenoidSet.vi"("error in (no error)"=w369, "Value"=WPI_SolenoidValue."On", "SolenoidDevRef"=w372) -> ("error out"=w368:errorcluster, "SolenoidDevRef"=w371:T30)  [unwired: 7 in]
                n151 = Wait (ms)(milliseconds to wait=w366) -> ()  [unwired: 1 out]
              }
              frame #2 {
                # "Retract Shooter"
                n152 = call-poly <vilib>:"WPI_SolenoidSet.vi"("error in (no error)"=w377, "Value"=WPI_SolenoidValue."Off", "SolenoidDevRef"=w378) -> ("error out"=w376:errorcluster)  [unwired: 7 in, 1 out]
                n153 = Wait (ms)(milliseconds to wait=w373) -> ()  [unwired: 1 out]
              }
              frame #3 {
                # "Close Claw"
                n154 = call-poly <vilib>:"WPI_SolenoidSet.vi"("error in (no error)"=w381, "Value"=WPI_SolenoidValue."Off", "SolenoidDevRef"=w379) -> ()  [unwired: 7 in, 2 out]
              }
            }
          }
        }
      }
      frame True {
      }
    }
    n155 = global write "Global Variables.vi" "Fire Ready"(w299) -> ()
  }
  n156 = call <vilib>:"WPI_SwitchRefNum Registry Get.vi"("refnum name"=T1 "Lock Disengaged" ("Device Name")) -> ("error out"=w28:errorcluster, "SwitchDevRef"=w35:T33)  [unwired: 9 in]
  n157 = call <vilib>:"WPI_MotorControlRefNum Registry Get.vi"("refnum name"=T1 "Arm Motor - Closed Loop Control" ("Device Name")) -> ("error out"=w34:errorcluster, "MotorControlDevRef"=w33:T10)  [unwired: 9 in]
  n158 = call <vilib>:"WPI_AnalogChannelRefNum Registry Get.vi"("refnum name"=T1 "Analog Arm Position Sensor" ("Device Name")) -> ("error out"=w31:errorcluster, "AIDeviceRef"=w32:T24)  [unwired: 9 in]
  n159 = call <vilib>:"WPI_SolenoidRefNum Registry Get.vi"("refnum name"=T1 "PCM - Arm Lock" ("Device Name")) -> ("error out"=w26:errorcluster, "SolenoidDevRef"=w27:T30)  [unwired: 9 in]
  n160 = while {
    tunnel: w35 -> [w406]
    tunnel: w34 -> [w405]
    tunnel: w33 -> [w404]
    tunnel: w32 -> [w400]
    tunnel: w31 -> [w387]
    tunnel: w28 -> [w403]
    tunnel: w27 -> [w402]
    tunnel: w26 -> [w401]
    stop <- FALSE stop-if-true
    # "Make it 'False' if unlocked"
    # "Returns 'True' if unlocked"
    # "Set Arm Lock"
    # "Arm Control"
    n161 = call <vilib>:"WPI_SwitchGetLimitValue.vi"("error in (no error)"=w403, "SwitchDevRef"=w406) -> ("Switch Pressed"=w383:bool)  [unwired: 7 in, 2 out]
    n162 = Not(x=w383) -> (.not. x?=w389:bool)
    n163 = global read "Global Variables.vi" "Arm Control"() -> (w407:T36)
    n164 = call-poly <vilib>:"NT Write Value.vi"("Boolean"=w383, "Name"="Arm Unlocked?") -> ()  [unwired: 9 in, 1 out]
    n165 = Unbundle By Name(w407) -> ("Arm Mode"=w382:T35)
    n166 = call "Arm - In Position Detector.vi"("error in (no error)"=w387, "Current Arm Mode"=w382, "AIDeviceRef"=w400) -> ("Current Angle"=w384:dbl, "Set Angle"=w385:dbl, "Disable Motor"=w388:bool, "Set Lock"=w386:bool)  [unwired: 4 in, 1 out]
    n167 = Equal?(x=w382, y=Arm_Mode_TypeDef."Disabled") -> (x = y?=w393:bool)
    n168 = Select(t=WPI_SolenoidValue."Forward" ("Value"), s=w386, f=WPI_SolenoidValue."Reverse" ("Value")) -> (s? t:f=w392:T32)
    n169 = Compound Arithmetic op=OR(w393, w389, w388) -> (w395:bool)
    n170 = call-poly <vilib>:"WPI_SolenoidSet.vi"("error in (no error)"=w401, "Value"=w392, "SolenoidDevRef"=w402) -> ()  [unwired: 7 in, 2 out]
    n171 = call "Falling Edge Detector.vi"("Input"=w395) -> ("Falling Edge Detected"=w398:bool)
    n172 = case shown="False" w395 {
      tunnel: w405 -> [w423 w432]
      tunnel: w404 -> [w424 w430]
      tunnel: w385 -> [w428 _]
      tunnel: w384 -> [w427 _]
      tunnel: w398 -> [w425 _]
      frame False {
        # "Arm Motor Enabled"
        n173 = call "Get NT PID Parameter.vi"("NT Path"="/Robot Parameters/Arm Parameters/Arm Motor PID Gains") -> ("PID Gains"=w420:T28)
        n174 = call-poly <vilib>:"PID.vi"("reinitialize? (F)"=w425, "output range"=cluster{"output high":dbl, "output low":dbl} {"output high"=1.0, "output low"=-1.0}, "PID gains"=w420, "process variable"=w427, "setpoint"=w428) -> ("output"=w421:dbl)  [unwired: 5 in, 1 out]
        n175 = call <vilib>:"WPI_CANTalonSRX_ChangeMode.vi"("error in (no error)"=w423, "Output"=w421, "Control Mode"=WPI_CANTalonSRX_APIControlMode."Percent VBus", "CAN Talon SRX Ref"=w424) -> ()  [unwired: 6 in, 2 out]
      }
      frame True {
        # "Arm Motor Disabled"
        n176 = call <vilib>:"WPI_CANTalonSRX_ChangeMode.vi"("error in (no error)"=w432, "Output"=0.0, "Control Mode"=WPI_CANTalonSRX_APIControlMode."Percent VBus", "CAN Talon SRX Ref"=w430) -> ()  [unwired: 6 in, 2 out]
      }
    }
    n177 = case shown="\"Cross Defense\"" w382 {
      tunnel: ["Invalid" "Disabled" "Locked" "Shoot Batter" "Shoot Close" "Cross Defense" "Human Player Load" "Low Bar / Goal" "Manual"] -> w396
      frame "Unknown", Default {
      }
      frame "Disabled" {
      }
      frame "Locked" {
      }
      frame "Shoot Batter" {
      }
      frame "Shoot Close" {
      }
      frame "Cross Defense" {
      }
      frame "Human Player Load" {
      }
      frame "Low Bar / Goal" {
      }
      frame "Manual" {
      }
    }
    n178 = Wait (ms)(milliseconds to wait=u32 20) -> ()  [unwired: 1 out]
    n179 = global write "Global Variables.vi" "Current Arm Mode"(w382) -> ()
    n180 = call-poly <vilib>:"NT Write Value.vi"("String"=w396, "Name"="Arm - Mode") -> ()  [unwired: 9 in, 1 out]
  }
  n181 = while {
    stop <- FALSE stop-if-true
    # "Operator Interface Control Board"
    n182 = global read "Global Variables.vi" "Fire Ready"() -> (w447:bool)
    n183 = global read "Global Variables.vi" "Arm Mode LEDs"() -> (w444:T39)
    n184 = Unbundle By Name(w444) -> ("Shoot Batter"=w443:bool, "Shoot Close"=w442:bool, "Shoot Far"=w441:bool, "Human Player Load"=w440:bool, "Low Bar / Goal"=w439:bool, "Manual"=w438:bool)
    n185 = Bundle By Name(cluster=T38 {"LED 0"=FALSE, "LED 1"=FALSE, "LED 2"=FALSE, "LED 3"=FALSE, "LED 4"=FALSE, "LED 5"=FALSE, "LED 6"=FALSE, "LED 7"=FALSE, "LED 8"=FALSE, "LED 9"=FALSE, "LED 10"=FALSE, "LED 11"=FALSE, "LED 12"=FALSE, "LED 13"=FALSE, "LED 14"=FALSE, "LED 15"=FALSE} ("LED Outputs"), "LED 0"=w447, "LED 1"=w443, "LED 2"=w442, "LED 3"=w441, "LED 4"=w440, "LED 5"=w439, "LED 6"=w438) -> (w445:T38)
    n186 = call "OICB - Set PWM.vi"("PWM Outputs"=T37 {"PWM 0"=0, "PWM 1"=0, "PWM 2"=0, "PWM 3"=0, "PWM 4"=0, "PWM 5"=0, "PWM 6"=0, "PWM 7"=0, "PWM 8"=0, "PWM 9"=0, "PWM 10"=0}) -> ()  [unwired: 10 in, 1 out]
    n187 = call "OICB - Get Switches.vi"() -> ("Switch Inputs"=w448:T26)  [unwired: 10 in, 1 out]
    n188 = call "OICB - Get Analog.vi"() -> ("Analog"=w434:T40)  [unwired: 10 in, 1 out]
    n189 = call "OICB - Set LED's.vi"("LED Outputs"=w445) -> ()  [unwired: 10 in, 1 out]
    n190 = global write "Global Variables.vi" "Analog Inputs"(w434) -> ()
    n191 = Wait (ms)(milliseconds to wait=u32 20) -> ()  [unwired: 1 out]
    n192 = Unbundle By Name(w434) -> ("ANA 0"=w435:u8)
    n193 = call "Autonomous - Get Mode.vi"("Autonomous Selector Value"=w435) -> ("Autonomous Mode"=w433:T41)  [unwired: 1 in]
    n194 = global write "Global Variables.vi" "Autonomous Mode"(w433) -> ()
    n195 = global write "Global Variables.vi" "Switch Inputs"(w448) -> ()
    n196 = call-poly <vilib>:"NT Write Value.vi"("Numeric"=w433, "Name"="Autonomous Mode") -> ()  [unwired: 9 in, 1 out]
  }
